vi "日期范围生成.vi"(7 "最小查询单位":enum16{"最小查询单位：天", "最小查询单位：月", "最小查询单位：年"}(ring), 8 "+日期？":bool=TRUE, 9 "日":u16, 10 "月":u16, 11 "年":u16) -> (0 "日期-大的":string, 3 "日期-小的":string)   [LabVIEW 2013]
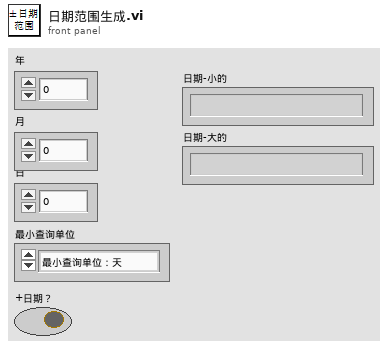
[diagram p1: front panel]
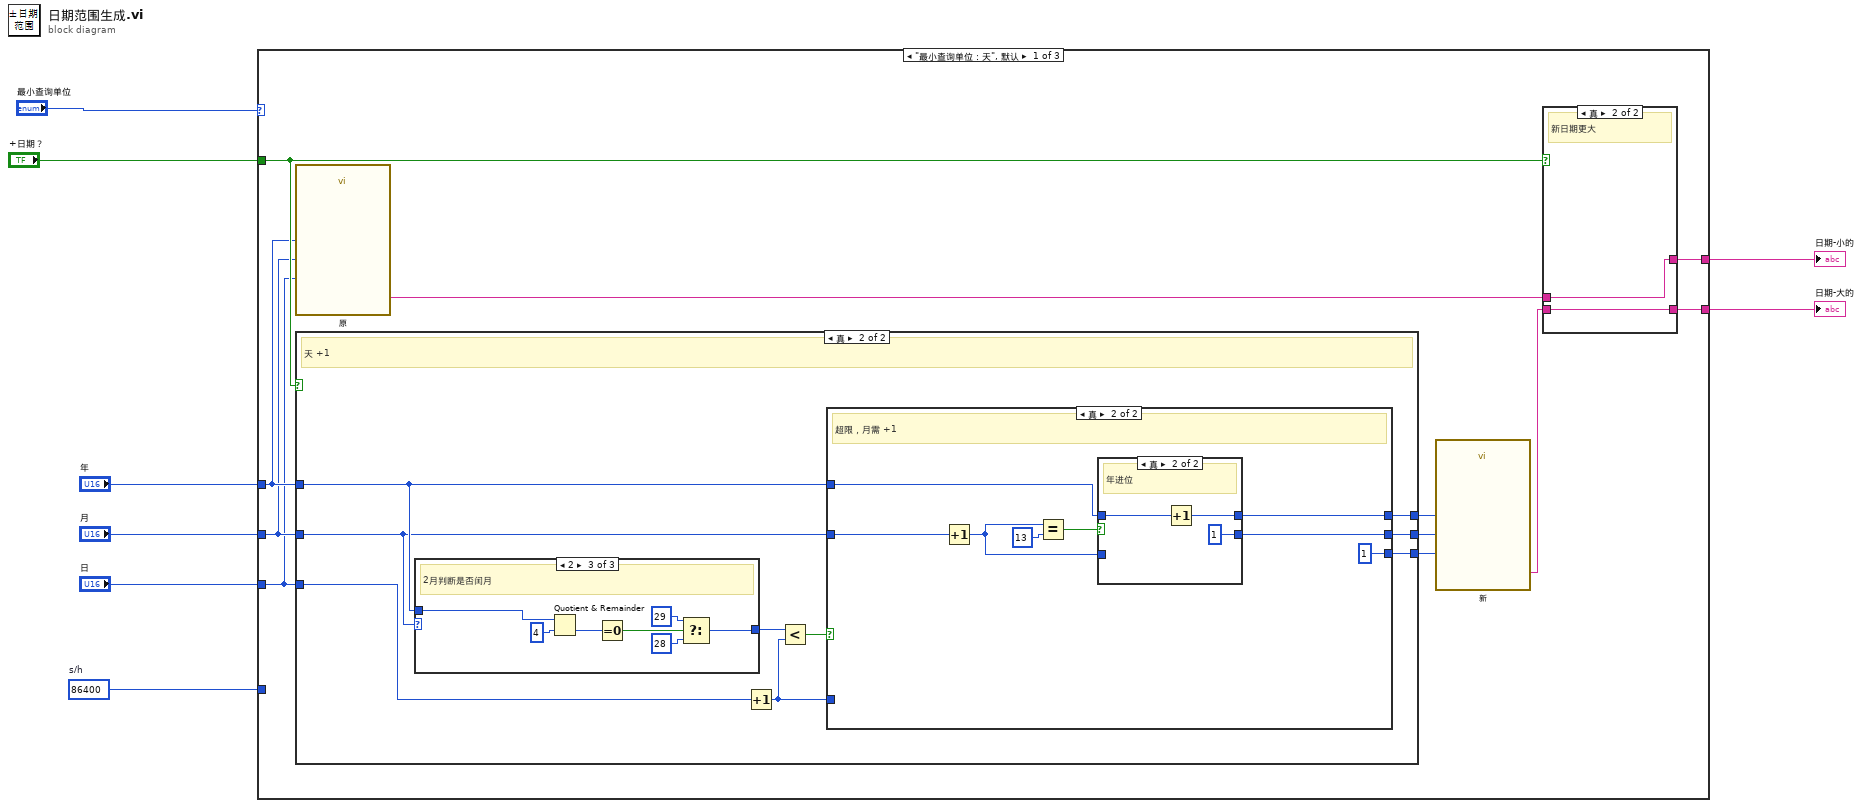
[diagram p0: block diagram]
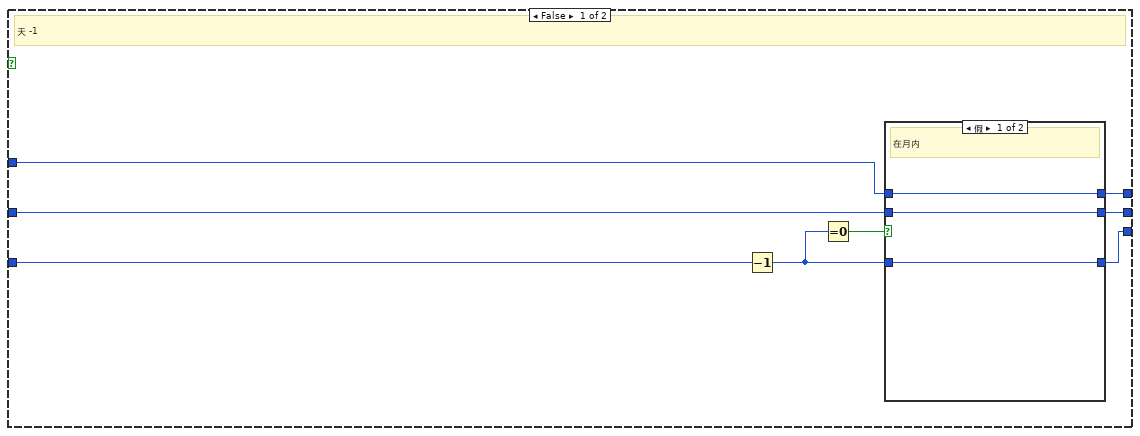
[diagram p2: hidden frame]
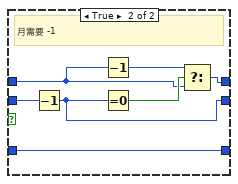
[diagram p3: hidden frame]
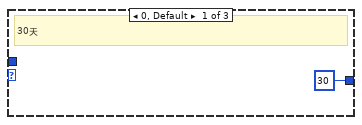
[diagram p6: hidden frame]
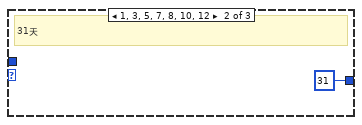
[diagram p7: hidden frame]
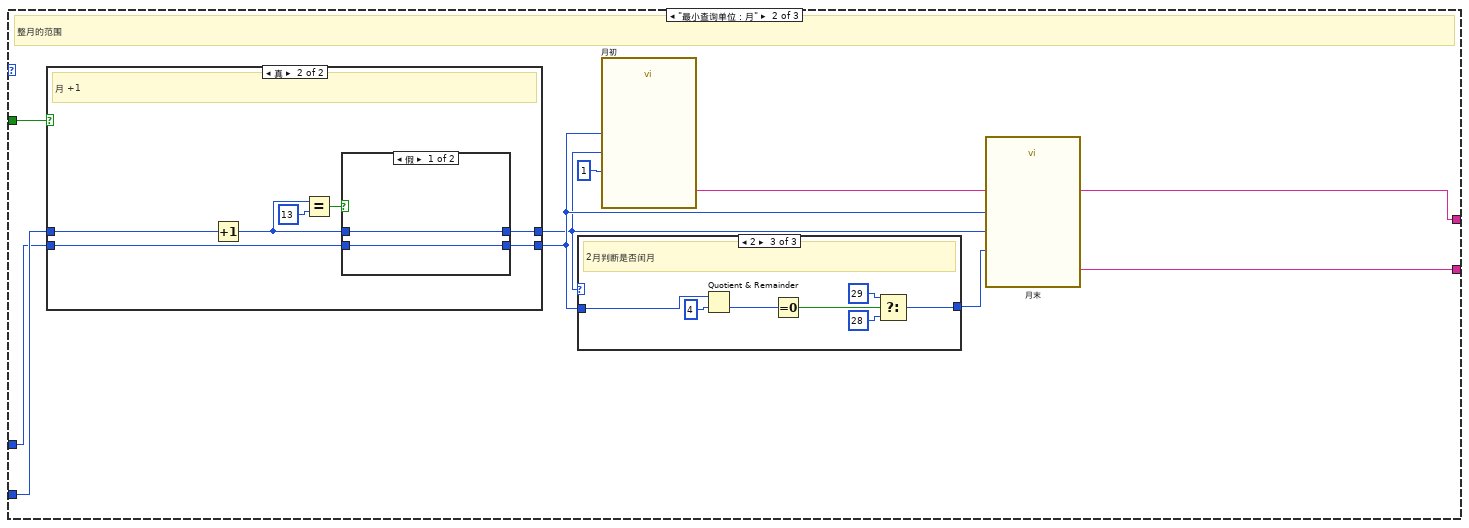
[diagram p9: hidden frame]
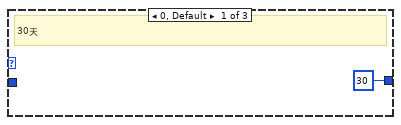
[diagram p10: hidden frame]
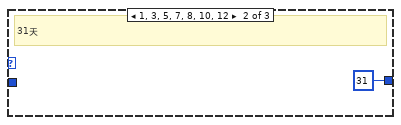
[diagram p11: hidden frame]
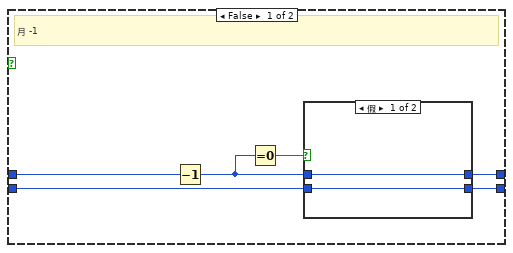
[diagram p12: hidden frame]
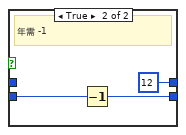
[diagram p13: hidden frame]
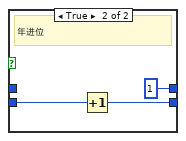
[diagram p14: hidden frame]
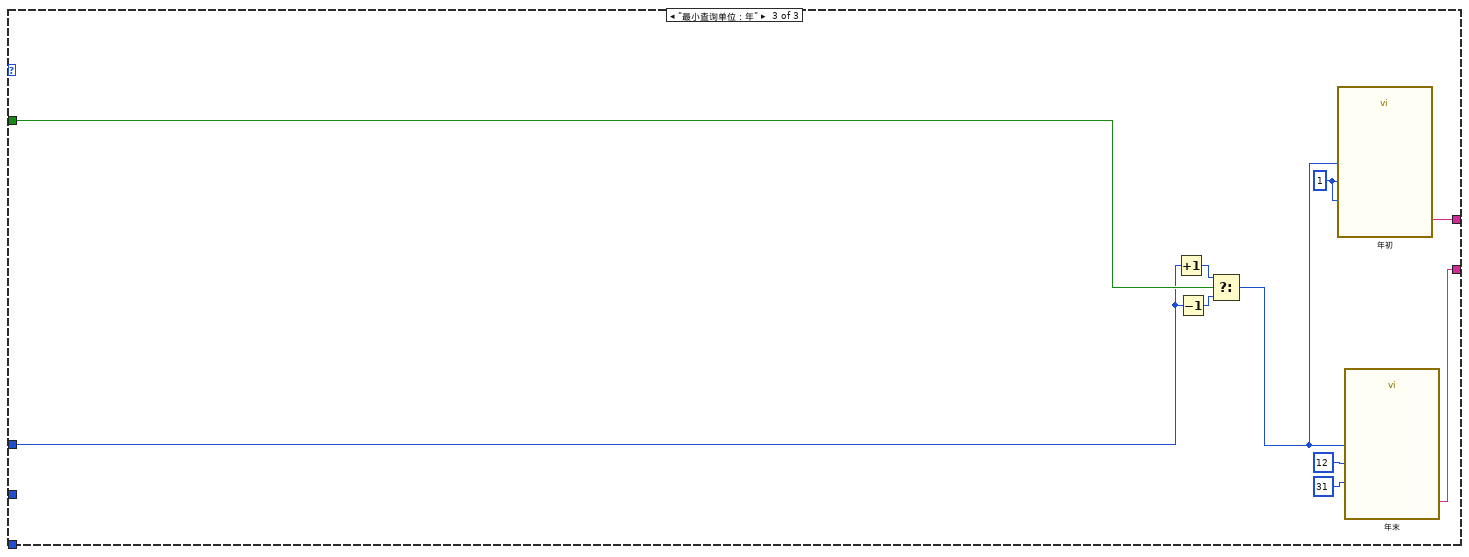
[diagram p15: hidden frame]
diagram:
  w4 = 86400  # s/h
  n1 = case shown="\"最小查询单位：天\", 默认" "最小查询单位" {
    tunnel: "年" -> [w11 w82 w118]
    tunnel: "月" -> [w10 w83 _]
    tunnel: "日" -> [w9 _ _]
    tunnel: "+日期？" -> [w15 w84 w121]
    tunnel: w4 -> [_ _ _]
    tunnel: [w17 w77 w123] -> w3
    tunnel: [w16 w76 w122] -> w2
    frame "最小查询单位：天", Default {
      n2 = call "原"("年"=w11, "月"=w10, "日"=w9) -> ("Result"=w18:string)  [unwired: 11 in, 1 out]
      n3 = case shown="真" w15 {
        tunnel: w9 -> [w27 w46]
        tunnel: w11 -> [w24 w43]
        tunnel: w10 -> [w25 w38]
        tunnel: [w20 w42] -> w14
        tunnel: [w21 w41] -> w13
        tunnel: [w22 w40] -> w12
        frame False {
          # "天 -1"
          n4 = Decrement(x=w27) -> (x-1=w23:u16)
          n5 = Equal To 0?(x=w23) -> (x = 0?=w26:bool)
          n6 = case shown="假" w26 {
            tunnel: w25 -> [w29 w37]
            tunnel: w24 -> [w30 w33]
            tunnel: w23 -> [w28 w36]
            tunnel: [w28 w36] -> w22
            tunnel: [w29 w35] -> w21
            tunnel: [w30 w31] -> w20
            frame False {
              # "在月内"
            }
            frame True {
              # "月需要 -1"
              n7 = Decrement(x=w37) -> (x-1=w35:u16)
              n8 = Decrement(x=w33) -> (x-1=w32:u16)
              n9 = Equal To 0?(x=w35) -> (x = 0?=w34:bool)
              n10 = Select(t=w32, s=w34, f=w33) -> (s? t:f=w31:u16)
            }
          }
        }
        frame True {
          # "天 +1"
          n11 = case shown="2" w38 {
            tunnel: w43 -> [_ _ w69]
            tunnel: [u16 30 ("y") u16 31 ("y") w65] -> w45
            frame 0, Default {
              # "30天"
            }
            frame 1, 3, 5, 7, 8, 10, 12 {
              # "31天"
            }
            frame 2 {
              # "2月判断是否闰月"
              n12 = Quotient & Remainder(x=w69, y=u16 4) -> (floor(x/y)=w71:u16)  [unwired: 1 out]
              n13 = Equal To 0?(x=w71) -> (x = 0?=w68:bool)
              n14 = Select(t=u16 29 ("y"), s=w68, f=u16 28 ("y")) -> (s? t:f=w65:u16)
            }
          }
          n15 = Increment(x=w46) -> (x+1=w39:u16)
          n16 = Less?(x=w45, y=w39) -> (x < y?=w44:bool)
          n17 = case shown="真" w44 {
            tunnel: w38 -> [w48 w57]
            tunnel: w43 -> [w49 w56]
            tunnel: [w49 w55] -> w42
            tunnel: [w48 w54] -> w41
            tunnel: [w47 u16 1 ("y")] -> w40
            tunnel: w39 -> [w47 _]
            frame False {
              # "在月内"
            }
            frame True {
              # "超限，月需 +1"
              n18 = Increment(x=w57) -> (x+1=w50:u16)
              n19 = Equal?(x=w50, y=u16 13) -> (x = y?=w51:bool)
              n20 = case shown="真" w51 {
                tunnel: w56 -> [w59 w62]
                tunnel: [w59 w61] -> w55
                tunnel: [w58 u16 1 ("y")] -> w54
                tunnel: w50 -> [w58 _]
                frame False {
                }
                frame True {
                  # "年进位"
                  n21 = Increment(x=w62) -> (x+1=w61:u16)
                }
              }
            }
          }
        }
      }
      n22 = call "新"("年"=w14, "月"=w13, "日"=w12) -> ("Result"=w19:string)  [unwired: 11 in, 1 out]
      n23 = case shown="真" w15 {
        tunnel: w19 -> [w72 w74]
        tunnel: w18 -> [w73 w75]
        tunnel: [w72 w75] -> w17
        tunnel: [w73 w74] -> w16
        frame False {
          # "原日期更大"
        }
        frame True {
          # "新日期更大"
        }
      }
    }
    frame "最小查询单位：月" {
      # "整月的范围"
      n24 = case shown="真" w84 {
        tunnel: w83 -> [w99 w111]
        tunnel: w82 -> [w97 w108]
        tunnel: [w96 w107] -> w80
        tunnel: [w95 w106] -> w79
        frame False {
          # "月 -1"
          n25 = Decrement(x=w99) -> (x-1=w94:u16)
          n26 = Equal To 0?(x=w94) -> (x = 0?=w98:bool)
          n27 = case shown="假" w98 {
            tunnel: w97 -> [w101 w104]
            tunnel: [w101 w103] -> w96
            tunnel: [w100 u16 12 ("y")] -> w95
            tunnel: w94 -> [w100 _]
            frame False {
            }
            frame True {
              # "年需 -1"
              n28 = Decrement(x=w104) -> (x-1=w103:u16)
            }
          }
        }
        frame True {
          # "月 +1"
          n29 = Increment(x=w111) -> (x+1=w105:u16)
          n30 = Equal?(x=w105, y=u16 13) -> (x = y?=w109:bool)
          n31 = case shown="假" w109 {
            tunnel: w108 -> [w113 w116]
            tunnel: [w113 w115] -> w107
            tunnel: [w112 u16 1 ("y")] -> w106
            tunnel: w105 -> [w112 _]
            frame False {
            }
            frame True {
              # "年进位"
              n32 = Increment(x=w116) -> (x+1=w115:u16)
            }
          }
        }
      }
      n33 = case shown="2" w79 {
        tunnel: w80 -> [_ _ w91]
        tunnel: [u16 30 ("y") u16 31 ("y") w87] -> w78
        frame 0, Default {
          # "30天"
        }
        frame 1, 3, 5, 7, 8, 10, 12 {
          # "31天"
        }
        frame 2 {
          # "2月判断是否闰月"
          n34 = Quotient & Remainder(x=w91, y=u16 4) -> (floor(x/y)=w93:u16)  [unwired: 1 out]
          n35 = Equal To 0?(x=w93) -> (x = 0?=w90:bool)
          n36 = Select(t=u16 29 ("y"), s=w90, f=u16 28 ("y")) -> (s? t:f=w87:u16)
        }
      }
      n37 = call "月初"("年"=w80, "月"=w79, "日"=u16 1 ("y")) -> ("Result"=w77:string)  [unwired: 11 in, 1 out]
      n38 = call "月末"("年"=w80, "月"=w79, "日"=w78) -> ("Result"=w76:string)  [unwired: 11 in, 1 out]
    }
    frame "最小查询单位：年" {
      w126 = u16 1 ("年")
      n39 = Increment(x=w118) -> (x+1=w120:u16)
      n40 = Decrement(x=w118) -> (x-1=w117:u16)
      n41 = Select(t=w120, s=w121, f=w117) -> (s? t:f=w119:u16)
      n42 = call "年初"("年"=w119, "月"=w126, "日"=w126) -> ("Result"=w123:string)  [unwired: 11 in, 1 out]
      n43 = call "年末"("年"=w119, "月"=u16 12 ("年"), "日"=u16 31 ("年")) -> ("Result"=w122:string)  [unwired: 11 in, 1 out]
    }
  }
  "日期-小的" <- w3
  "日期-大的" <- w2
